vi "PTSequencer.destructor.vi"(0 "i ref in":refnum<vi>, 5 "error in (no error)":errorcluster) -> (19 "error out":errorcluster)   [LabVIEW 2014, in "PTSequencer.lvlib"]
uses:
  PTSequencer.lvlib
  CSCore/BaseProcess/BaseProcess.lvlib
  CSCore/BaseSM/BaseSM.lvlib
  CSCore/BaseGUI/BaseGUI.lvlib
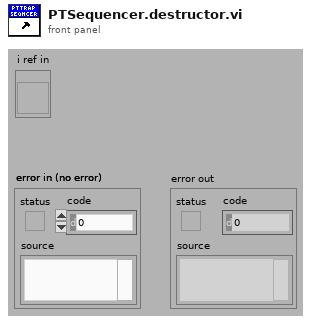
[diagram p1: front panel]
types:
  T1 = enum16{"SetAttribute", "GetAttribute", "CreateAttribute", "DestroyAttribute", "DestroyAllAtributes"}
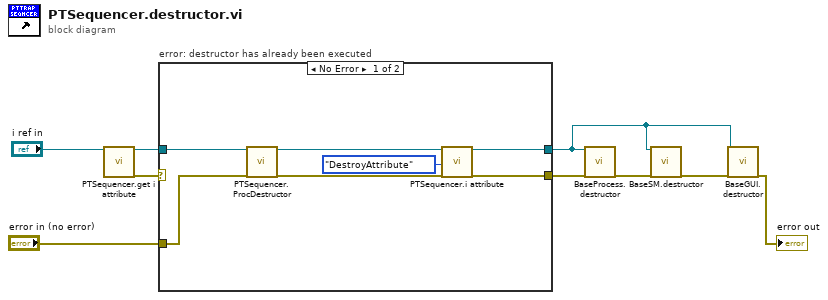
[diagram p0: block diagram]
diagram:
  n1 = call "PTSequencer.get i attribute.vi"("i ref in"="i ref in") -> ("i ref out"=w7:refnum<vi>, "error out"=w8:errorcluster)  [unwired: 16 in, 1 out]
  n2 = case "error: destructor has already been executed" shown="No Error" w8 {
    selector: w8 -> [_ w17]
    tunnel: w7 -> [w13 w18]
    tunnel: [w15 w18] -> w2
    tunnel: [w14 w17] -> w6
    tunnel: "error in (no error)" -> [w12 _]
    frame No Error {
      n3 = call "PTSequencer.ProcDestructor.vi"("i ref in"=w13, "error in (no error)"=w12) -> ("i ref out"=w10:refnum<vi>, "error out"=w11:errorcluster)  [unwired: 16 in]
      n4 = call "PTSequencer.i attribute.vi"("VI Refnum"=w10, "Action"=T1."DestroyAttribute", "error in (no error)"=w11) -> ("VI Refnum out"=w15:refnum<vi>, "error out"=w14:errorcluster)  [unwired: 14 in, 1 out]
    }
    frame Error {
    }
  }
  n5 = call "BaseProcess.destructor.vi"("i ref in"=w2, "error in (no error)"=w6) -> ("error out"=w4:errorcluster)  [unwired: 17 in]
  n6 = call "BaseSM.destructor.vi"("i ref in"=w2, "error in (no error)"=w4) -> ("error out"=w3:errorcluster)  [unwired: 17 in]
  n7 = call "BaseGUI.destructor.vi"("i ref in"=w2, "error in (no error)"=w3) -> ("error out"=→"error out":errorcluster)  [unwired: 17 in]
